vi "DigitalOutput-Make tasks.vi"(3 "Timestamp lines":tag[](array[tag]), 4 "DO timestamp lines":tag[](array[tag]), 5 "Output Lines":tag[](array[tag])) -> (0 "TS only":refnum<k21>[](array[refnum]), 1 "line+TS":refnum<k21>[](array[refnum]), 2 "line only":refnum<k21>[](array[refnum]))   [LabVIEW 2015]
doc: "Turns physical line names (e.g. Dev1/port0/line0) into digital output tasks.\n\nAlso, creates another set of tasks with timestamp lines appended."
uses:
  <vilib>/DAQmx/create/channels.llb/DAQmx Create Channel (DO-Digital Output).vi
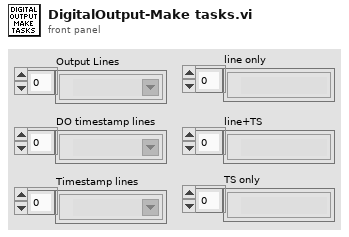
[diagram p1: front panel]
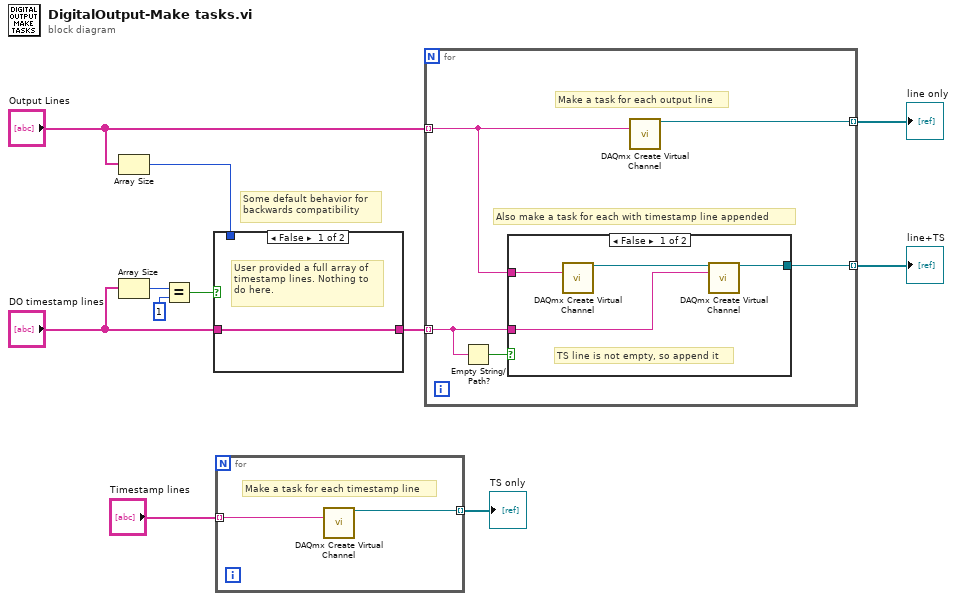
[diagram p0: block diagram]
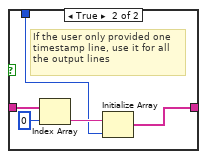
[diagram p2: hidden frame]
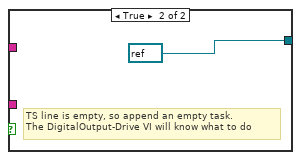
[diagram p3: hidden frame]
diagram:
  # "Some default behavior for\nbackwards compatibility"
  n1 = Array Size(array="Output Lines") -> (size(s)=w3:i32)
  n2 = Array Size(array="DO timestamp lines") -> (size(s)=w7:i32)
  n3 = Equal?(x=w7, y=1) -> (x = y?=w5:bool)
  n4 = case shown="False" w5 {
    tunnel: [w12 w13] -> w9
    tunnel: "DO timestamp lines" -> [w12 w17]
    tunnel: w3 -> [_ w14]
    frame False {
      # "User provided a full array of\ntimestamp lines. Nothing to\ndo here."
    }
    frame True {
      # "If the user only provided one\ntimestamp line, use it for all\nthe output lines"
      n5 = Index Array(array=w17, index=0) -> (element=w15:tag)
      n6 = Initialize Array(w15, w14) -> (w13:tag[])
    }
  }
  n7 = for {
    tunnel: "Timestamp lines" -> [w18] mode=indexing
    tunnel: [w19] -> w1 mode=indexing
    # "Make a task for each timestamp line"
    n8 = call-poly <vilib>:"DAQmx Create Virtual Channel.vi"("lines"=w18) -> ("task out"=w19:refnum<k21>)  [unwired: 13 in, 1 out]
  }
  "TS only" <- w1
  n9 = for {
    tunnel: "Output Lines" -> [w23] mode=indexing
    tunnel: w9 -> [w21] mode=indexing
    tunnel: [w24] -> w11 mode=indexing
    tunnel: [w22] -> w10 mode=indexing
    # "Also make a task for each with timestamp line appended"
    # "Make a task for each output line"
    n10 = Empty String/Path?(string/path=w21) -> (empty?=w20:bool)
    n11 = case shown="False" w20 {
      tunnel: w23 -> [w27 _]
      tunnel: [w26 refnum<k21> refnum ("task out")] -> w22
      tunnel: w21 -> [w25 _]
      frame False {
        # "TS line is not empty, so append it"
        n12 = call-poly <vilib>:"DAQmx Create Virtual Channel.vi"("lines"=w27) -> ("task out"=w28:refnum<k21>)  [unwired: 13 in, 1 out]
        n13 = call-poly <vilib>:"DAQmx Create Virtual Channel.vi"("task in"=w28, "lines"=w25) -> ("task out"=w26:refnum<k21>)  [unwired: 12 in, 1 out]
      }
      frame True {
        # "TS line is empty, so append an empty task.\nThe DigitalOutput-Drive VI will know what to do"
      }
    }
    n14 = call-poly <vilib>:"DAQmx Create Virtual Channel.vi"("lines"=w23) -> ("task out"=w24:refnum<k21>)  [unwired: 13 in, 1 out]
  }
  "line only" <- w11
  "line+TS" <- w10
